vi "Inicializar Fecha.vi"(8 "error in (no error)":errorcluster, 11 "FirstActor in":refnum<class "FirstActor.lvclass">) -> (0 "error out":errorcluster, 3 "FirstActor out":refnum<class "FirstActor.lvclass">)   [LabVIEW 2020, in "FirstActor.lvlib" / "FirstActor.lvclass"]
uses:
  FirstActor.lvclass
  FirstActor.lvclass/FirstActor.ctl
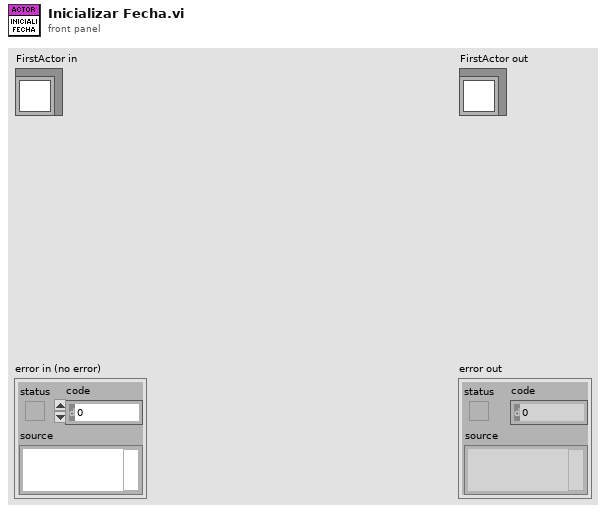
[diagram p1: front panel]
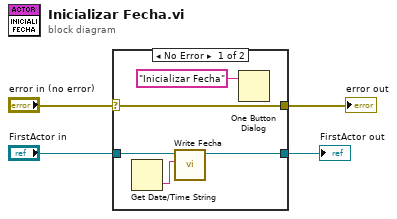
[diagram p0: block diagram]
diagram:
  n1 = case shown="No Error" "error in (no error)" {
    selector: "error in (no error)" -> [w9 w11]
    tunnel: [w9 w11] -> w3
    tunnel: [w6 w10] -> w1
    tunnel: "FirstActor in" -> [w7 w10]
    frame No Error {
      n2 = Get Date/Time String() -> (time string=w8:string)  [unwired: 3 in, 1 out]
      n3 = call "Write Fecha.vi"("Fecha"=w8, "FirstActor in"=w7) -> ("FirstActor out"=w6:refnum<class "FirstActor.lvclass">)  [unwired: 8 in, 1 out]
      n4 = One Button Dialog(message="Inicializar Fecha") -> ()  [unwired: 1 in, 1 out]
    }
    frame Error {
    }
  }
  "error out" <- w3
  "FirstActor out" <- w1
